vi "Add Event - Master.vi"(8 "error in (no error)":errorcluster, 10 "Event":T1, 11 "Controller in":refnum<class "Controller.lvclass">) -> (0 "error out":errorcluster, 3 "Controller out":refnum<class "Controller.lvclass">)   [LabVIEW 2019, in "Controller.lvlib" / "Controller.lvclass"]
uses:
  Controller.lvclass
  Sensors/Detector/Event.ctl
  Controller.lvclass/Controller.ctl
  Sensors/Detector/Muon Detector.lvclass
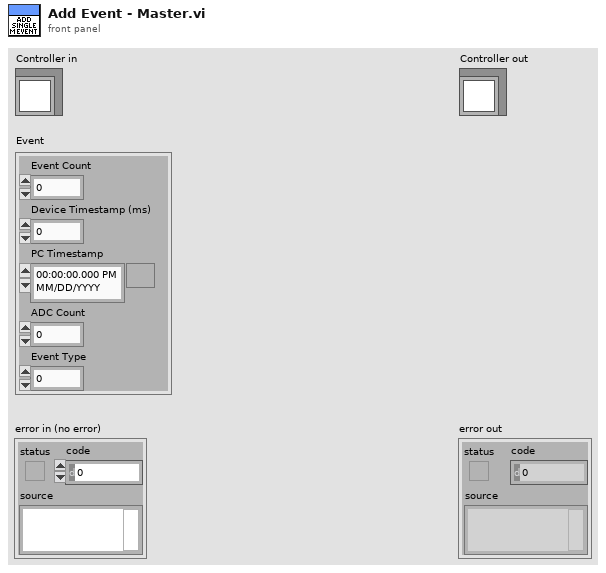
[diagram p1: front panel]
types:
  T1 = typedef "Muon Detector.lvclass/Event.ctl" = cluster{"Event Count":i32, "Device Timestamp (ms)":i32, "PC Timestamp":timestamp, "ADC Count":i32, "Event Type":u8}
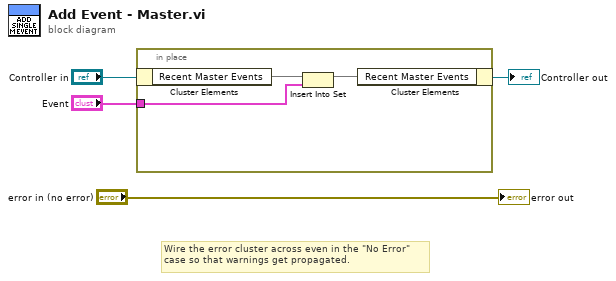
[diagram p0: block diagram]
diagram:
  # "Wire the error cluster across even in the \"No Error\"\ncase so that warnings get propagated."
  n1 = in-place {
    in-place-border: "Event" -> [w5]
    n2 = in-place-cluster #1("Controller in") -> ("Recent Master Events"=w7:set{T1})
    n3 = Insert Into Set(10:w5, 11:w7) -> (3:w6:set{T1})  [unwired: 1 out]
    n4 = in-place-cluster #1("Recent Master Events"=w6) -> (→"Controller out":refnum<class "Controller.lvclass">)
  }
  "error out" <- "error in (no error)"
